vi "ROI_Image_Determine Circles.vi"(8 "error in (no error)":errorcluster, 11 "Image in":T1) -> (0 "error out":errorcluster, 1 "N Circles":i32, 2 "Circle Data":T2(array[cluster]), 3 "Image out":T1)   [LabVIEW 2012]
uses:
  <vilib>/vision/Image Controls.llb/IMAQ Image.ctl
  FileIO/TypeDef - File Actions.ctl
  <vilib>/vision/NI_Vision_Development_Module.lvlib
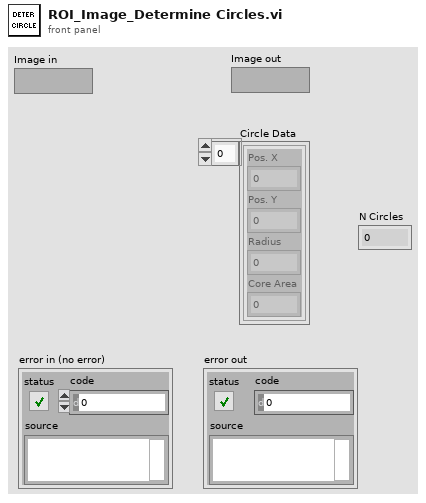
[diagram p1: front panel]
types:
  T1 = typedef "IMAQ Image.ctl" = refnum<image>
  T2 = cluster{"Pos. X":i32, "Pos. Y":i32, "Radius":i32, "Core Area":i32}[]
  T3 = typedef "TypeDef - File Actions.ctl" = enum16{"Read", "Write", "Get Current"}
  T4 = typedef "TypeDef - System Configuration.ctl" = cluster{"Results FilePath":path, "Analysis Parameters":cluster{"Threshold Range":cluster{"Lower Value":i32, "Upper Value":i32}, "Particle Erosion":cluster{"N Steps":u32}, "Feret Filter ":cluster{"Lower Value":dbl, "Upper Value":dbl}, "Circle Filter Diameter":cluster{"Min Radius":sgl, "Max Radius":sgl}}}
  T5 = cluster{"Pos. X":i32, "Pos. Y":i32, "Radius":i32, "Core Area":i32}
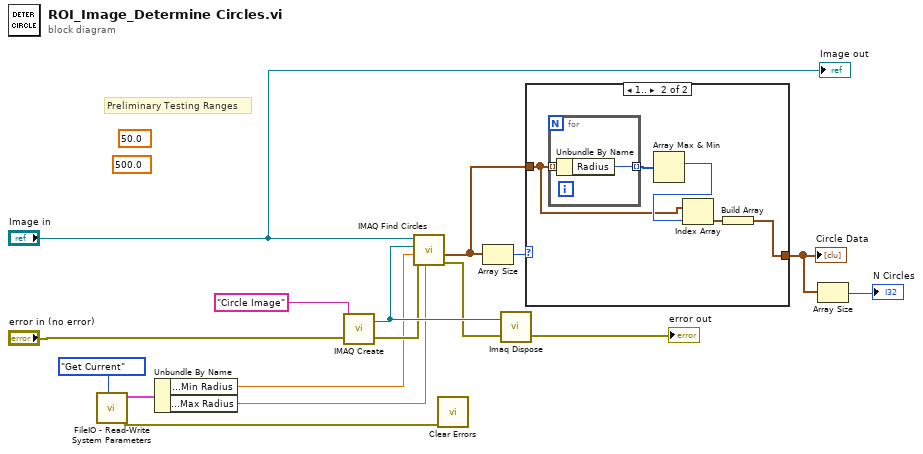
[diagram p0: block diagram]
diagram:
  (unwired) sgl 500.0 ("Max Radius")
  (unwired) sgl 50.0 ("Min Radius")
  # "Preliminary Testing Ranges"
  n1 = call "FileIO - Read-Write System Parameters.vi"("Action"=TypeDef_-_File_Actions."Get Current") -> ("error out"=w3:errorcluster, "HW Configuration (each Station)"=w4:T4)  [unwired: 9 in]
  n2 = Unbundle By Name(w4) -> ("Analysis Parameters.Circle Filter Diameter.Min Radius"=w2:sgl, "Analysis Parameters.Circle Filter Diameter.Max Radius"=w1:sgl)
  n3 = call "IMAQ Create"("Image Name"="Circle Image", "error in (no error)"="error in (no error)") -> ("New Image"=w15:T1, "error out"=w12:errorcluster)  [unwired: 2 in, 1 out]
  n4 = call "IMAQ Find Circles"("Max Radius"=w1, "error in (no error)"=w12, "Min Radius"=w2, "Image Dst"=w15, "Image Src"="Image in") -> ("error out"=w13:errorcluster, "Circles Data"=w11:T2)  [unwired: 5 out]
  n5 = call <vilib>:"Clear Errors.vi"("error in (no error)"=w3) -> ()  [unwired: 6 in, 1 out]
  n6 = Array Size(array=w11) -> (size(s)=w9:i32)
  n7 = call "Imaq Dispose"("Image"=w15, "error in (no error)"=w13) -> ("error out"=→"error out":errorcluster)  [unwired: 4 in]
  n8 = case shown="1.." w9 {
    tunnel: w11 -> [w17 w19]
    tunnel: [w17 w18] -> w6
    frame 0, Default {
      # "If no Circle data, just pass empty array"
    }
    frame 1.. {
      n9 = for {
        tunnel: w19 -> [w24] mode=indexing
        tunnel: [w23] -> w20 mode=indexing
        n10 = Unbundle By Name(w24) -> ("Radius"=w23:i32)
      }
      n11 = Array Max & Min(array=w20) -> (max index (indices)=w21:i32)  [unwired: 3 out]
      n12 = Index Array(array=w19, index=w21) -> (element=w22:T5)
      n13 = Build Array(w22) -> (w18:T2)
    }
  }
  "Circle Data" <- w6
  n14 = Array Size(array=w6) -> (size(s)=→"N Circles":i32)
  "Image out" <- "Image in"
